vi "Selector.vi"(7 "Group_Num":i32, 10 "Select":i32[](array[numeric]), 11 "X (input Data Array, 2D)":dbl[][](array[numeric])) -> (3 "SubArray":dbl[][](array[numeric]))   [LabVIEW 2014]
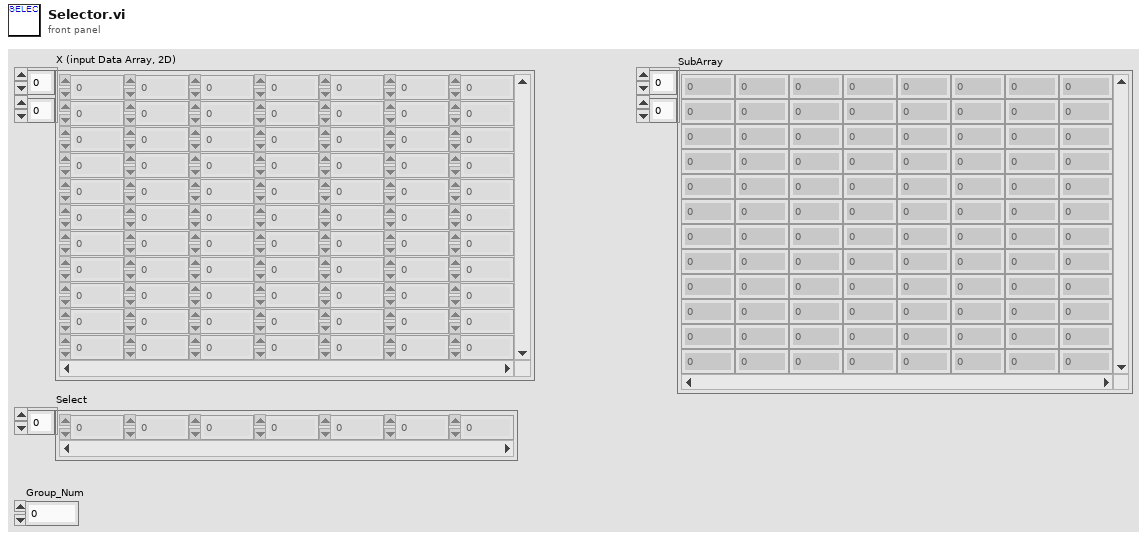
[diagram p1: front panel]
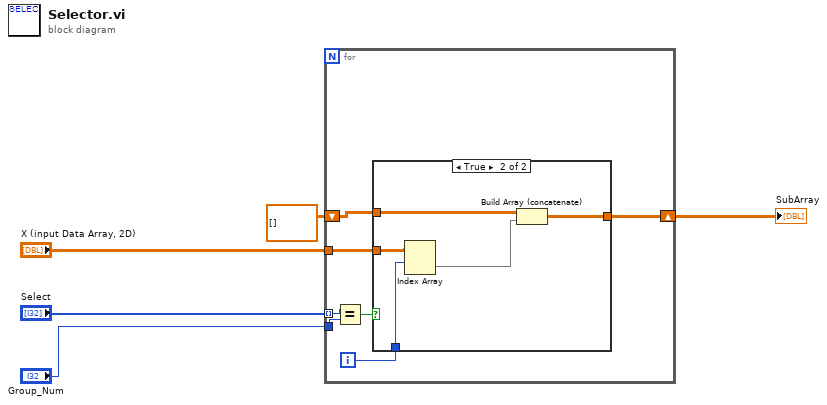
[diagram p0: block diagram]
diagram:
  n1 = for {
    tunnel: "Select" -> [w7] mode=indexing
    tunnel: "X (input Data Array, 2D)" -> [w12]
    shift-right: [w11] -> w3
    shift-left: dbl[][] [] -> [w10]
    tunnel: "Group_Num" -> [w6]
    i -> [w9]
    n2 = Equal?(x=w7, y=w6) -> (x = y?=w8:bool)
    n3 = case shown="True" w8 {
      tunnel: w12 -> [_ w18]
      tunnel: [w13 w16] -> w11
      tunnel: w10 -> [w13 w15]
      tunnel: w9 -> [_ w14]
      frame False {
      }
      frame True {
        n4 = Index Array(array=w18, index (row)=w14) -> (element=w17:dbl[])  [unwired: 1 in]
        n5 = Build Array (concatenate)(w15, w17) -> (w16:dbl[][])
      }
    }
  }
  "SubArray" <- w3
